vi "POST File.vi"(6 "server file name":string, 7 "file path":path, 8 "error in (no error)":errorcluster, 9 "buffer":string, 10 "relative URL":string, 11 "eLab in":refnum<class "PL eLabFTW Client.lvclass">) -> (0 "error out":errorcluster, 2 "response body":string, 3 "eLab out":refnum<class "PL eLabFTW Client.lvclass">)   [LabVIEW 2015, in "PL eLabFTW Client.lvclass"]
doc: "Performs POST request with the specified buffer or file and returns the response body."
uses:
  PL eLabFTW Client.lvclass
  <vilib>/httpClient/MultipartData.ctl
  PL eLabFTW Client.lvclass/PL eLabFTW Client.ctl
  <vilib>/httpClient/LabVIEWHTTPClient.lvlib
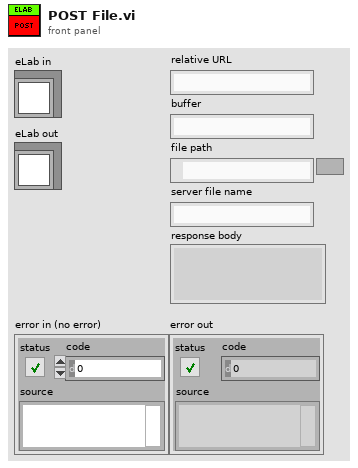
[diagram p1: front panel]
types:
  T1 = typedef "LabVIEWHTTPClient.lvlib/MultipartData.ctl" = cluster{"Name":string, "Value":string, "File":path, "Filename":string, "MIME type":string}
  T2 = typedef "LabVIEWHTTPClient.lvlib/ClientHandle.ctl" = refnum<k1>
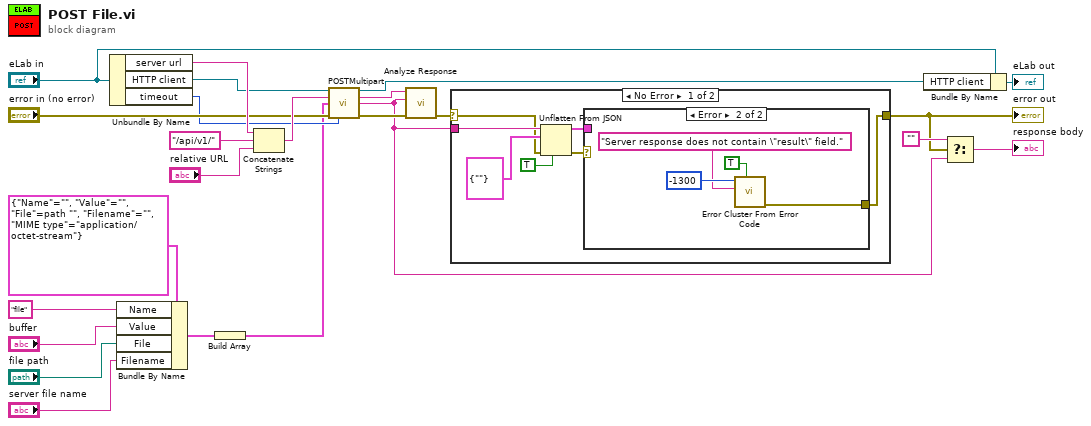
[diagram p0: block diagram]
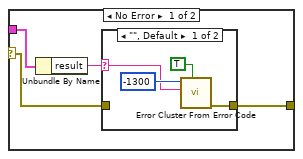
[diagram p2: hidden frame]
diagram:
  n1 = Unbundle By Name("eLab in") -> ("server url"=w24:string, "HTTP client"=w14:T2, "timeout"=w8:i32)
  n2 = Bundle By Name(cluster=T1 {"Name"="", "Value"="", "File"=path "", "Filename"="", "MIME type"="application/octet-stream"} ("Element"), "Name"="file", "Value"="buffer", "File"="file path", "Filename"="server file name") -> (w2:T1)
  n3 = Build Array(w2) -> (w1:T1[])
  n4 = Concatenate Strings(w24, "/api/v1/" ("string"), "relative URL") -> (w13:string)
  n5 = call <vilib>:"POSTMultipart.vi"("client handle"=w14, "url"=w13, "data"=w1, "error in (no error)"="error in (no error)", "timeout (10000)"=w8) -> ("client handle out"=w15:T2, "headers"=w10:string, "body"=w9:string, "error out"=w11:errorcluster)  [unwired: 7 in]
  n6 = call "Analyze Response.vi"("error in (no error)"=w11, "body"=w9, "headers"=w10) -> ("error out"=w17:errorcluster)  [unwired: 8 in]
  n7 = case shown="No Error" w17 {
    selector: w17 -> [w25 w45]
    tunnel: w9 -> [w31 _]
    tunnel: [w27 w45] -> w16
    frame No Error {
      n8 = Unflatten From JSON(JSON string=w31, type and defaults=cluster{"result":string} {"result"=""}, default null elements? (F)=TRUE, error in (no error)=w25) -> (value=w26:cluster{"result":string}, error out=w28:errorcluster)  [unwired: 3 in]
      n9 = case shown="Error" w28 {
        selector: w28 -> [w33 _]
        tunnel: [w32 w41] -> w27
        tunnel: w26 -> [w35 _]
        frame No Error {
          n10 = Unbundle By Name(w35) -> ("result"=w34:string)
          n11 = case shown="\"\", Default" w34 {
            selector: w34 -> [w37 _]
            tunnel: w33 -> [_ w40]
            tunnel: [w36 w40] -> w32
            frame "", Default {
              n12 = call <vilib>:"Error Cluster From Error Code.vi"("show call chain? (False)"=TRUE, "error message (\"\")"=w37, "error code (0)"=-1300) -> ("error out"=w36:errorcluster)  [unwired: 6 in]
            }
            frame "success" {
            }
          }
        }
        frame Error {
          n13 = call <vilib>:"Error Cluster From Error Code.vi"("show call chain? (False)"=TRUE, "error message (\"\")"="Server response does not contain \"result\" field." ("format string"), "error code (0)"=-1300) -> ("error out"=w41:errorcluster)  [unwired: 6 in]
        }
      }
    }
    frame Error {
    }
  }
  "error out" <- w16
  n14 = Bundle By Name(cluster="eLab in", "HTTP client"=w15) -> (→"eLab out":refnum<class "PL eLabFTW Client.lvclass">)
  n15 = Select(t="", s=w16, f=w9) -> (s? t:f=→"response body":string)
